vi "Set Instr Ident.vi"(10 "Instr Ident":string, 11 "CFG Base in":refnum<class "CFG Base.lvclass">) -> (3 "CFG Base out":refnum<class "CFG Base.lvclass">)   [LabVIEW 2023, in "HAL.lvlib" / "CFG Base.lvclass"]
uses:
  CFG Base.lvclass
  CFG Base.lvclass/CFG Base.ctl
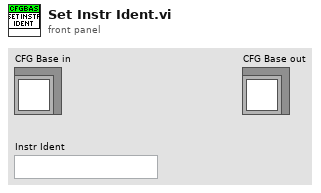
[diagram p1: front panel]
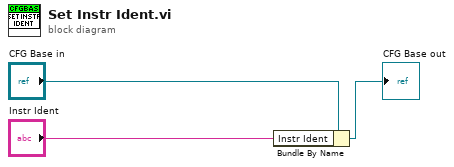
[diagram p0: block diagram]
diagram:
  n1 = Bundle By Name(cluster="CFG Base in", "Instr Ident"="Instr Ident") -> (→"CFG Base out":refnum<class "CFG Base.lvclass">)
